vi "Sort (single).vi"(8 "error in (no error)":errorcluster, 11 "XY-data":cluster{"X-array":dbl[], "Y-array":dbl[]}) -> (0 "error out":errorcluster, 3 "Sorted XY-data out":cluster{"X-array":dbl[], "Y-array":dbl[]} {"Y-array" format="%.2p"; "X-array" format="%.2p"})   [LabVIEW 2019, in "xy_utilities.lvlib"]
doc: "Sorts the input <b>XY-data</b> according to its x array.\n\nWire data to the data input to determine the polymorphic instance to use or manually select the instance."
uses:
  xy_utilities.lvlib
  _OpenG.lib/array/array.llb/Sort 1D Array (DBL)__ogtk.vi
  _OpenG.lib/array/array.llb/Reorder 1D Array2 (DBL)__ogtk.vi
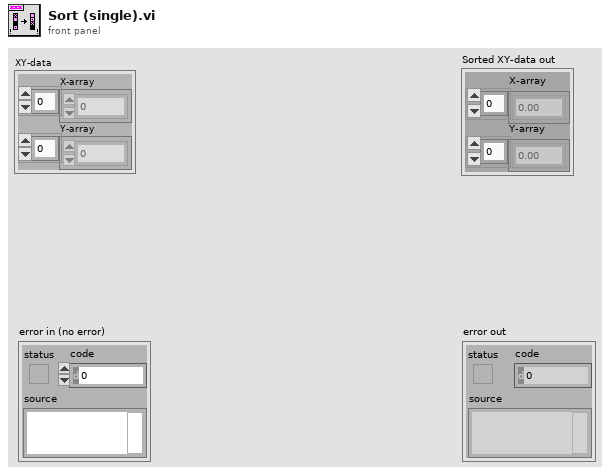
[diagram p1: front panel]
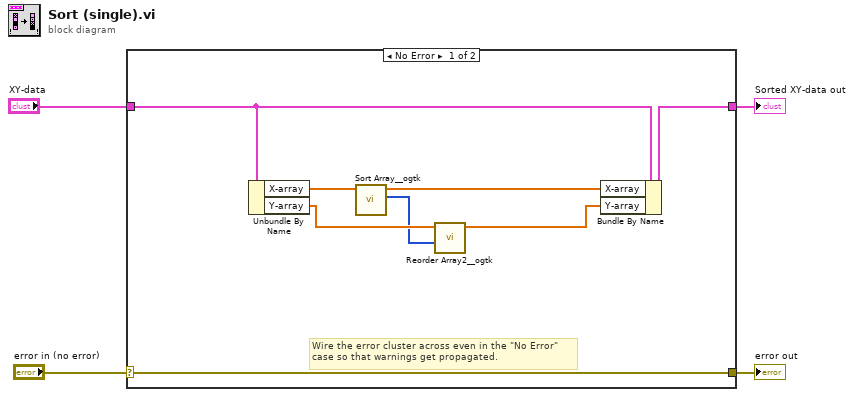
[diagram p0: block diagram]
diagram:
  n1 = case shown="No Error" "error in (no error)" {
    selector: "error in (no error)" -> [w12 w14]
    tunnel: [w12 w14] -> w3
    tunnel: "XY-data" -> [w11 w13]
    tunnel: [w10 w13] -> w1
    frame No Error {
      # "Wire the error cluster across even in the \"No Error\"\ncase so that warnings get propagated."
      n2 = Unbundle By Name(w11) -> ("X-array"=w9:dbl[], "Y-array"=w8:dbl[])
      n3 = call-poly "Sort Array__ogtk.vi"("Array in"=w9) -> ("Sorted Pointers"=w5:i32[], "Sorted Array out"=w7:dbl[])  [unwired: 9 in]
      n4 = call-poly "Reorder Array2__ogtk.vi"("indices"=w5, "array"=w8) -> ("reordered array"=w6:dbl[])  [unwired: 9 in]
      n5 = Bundle By Name(cluster=w11, "X-array"=w7, "Y-array"=w6) -> (w10:cluster{"X-array":dbl[], "Y-array":dbl[]})
    }
    frame Error {
    }
  }
  "error out" <- w3
  "Sorted XY-data out" <- w1
